vi "niDTS Comm String Flush Port.vi"(0 "Comm String Handle":T1, 7 "Read Data (F)":bool, 9 "Log Data (F)":bool, 11 "error in (no error)":errorcluster) -> (4 "Comm String Handle Out":T1, 6 "Response":string, 15 "error out":errorcluster)   [LabVIEW 2014, in "niDTS CommLib.lvlib"]
doc: "This sends the Command concatenated with the Args over the String Interface.\n\nInputs:\n* Command (Required): This is the command to be sent.\n* Args (Optional): Any arguments to be concatenated with the command.\n\nOutputs:\n* Response: Any data returned from the interface. Note that no data wil be returned if the flag Read Enabled is set to FALSE."
uses:
  niDTS CommLib.lvlib
  Includes/niDTS Comm String INC Handle.ctl
  Objects/String_class/niDTS Comm String.lvclass
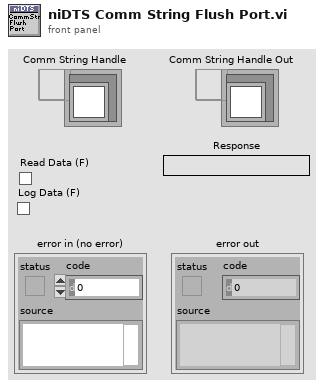
[diagram p1: front panel]
types:
  T1 = typedef "niDTS CommLib.lvlib/niDTS Comm String INC Handle.ctl" = refnum<data-value>
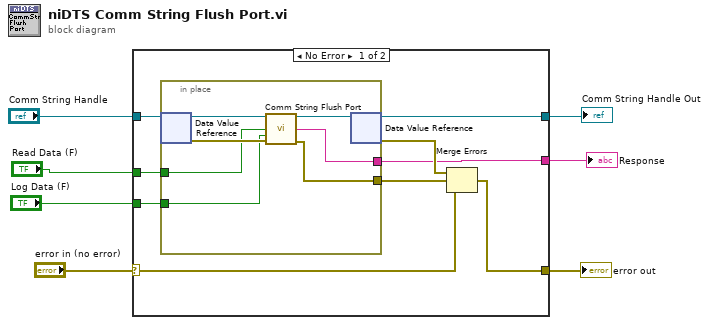
[diagram p0: block diagram]
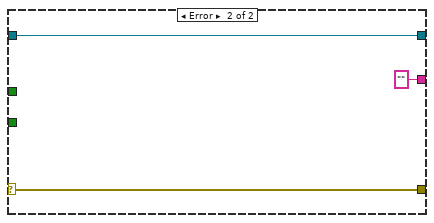
[diagram p2: hidden frame]
diagram:
  n1 = case shown="No Error" "error in (no error)" {
    selector: "error in (no error)" -> [w14 w26]
    tunnel: [w13 w26] -> w7
    tunnel: "Comm String Handle" -> [w16 w25]
    tunnel: [w12 w25] -> w4
    tunnel: [w10 "" ("Response")] -> w3
    tunnel: "Read Data (F)" -> [w9 _]
    tunnel: "Log Data (F)" -> [w8 _]
    frame No Error {
      n2 = in-place {
        in-place-border: [w20] -> w11
        in-place-border: [w19] -> w10
        in-place-border: w9 -> [w18]
        in-place-border: w8 -> [w17]
        n3 = in-place-dvr #1(w16) -> (w23:refnum<class "niDTS Comm String.lvclass">, w22:errorcluster)
        n4 = call-dynamic "Comm String Flush Port.vi"("niDTS Comm String in"=w23, "Read Data (F)"=w18, "Log Data (F)"=w17, "error in (no error)"=w22) -> ("niDTS Comm String out"=w21:refnum<class "niDTS Comm String.lvclass">, "Read Data"=w19:string, "error out"=w20:errorcluster)  [unwired: 9 in]
        n5 = in-place-dvr #1(w21) -> (w12:T1, w15:errorcluster)
      }
      n6 = Merge Errors(w15, w11, w14) -> (w13:errorcluster)
    }
    frame Error {
    }
  }
  "error out" <- w7
  "Comm String Handle Out" <- w4
  "Response" <- w3
